vi "V50_OfficeReport.vi"(1 "Enable":bool=TRUE, 2 "blockFabric":variant, 3 "blockRange":variant, 4 "blockResults":variant, 5 "blockSample":variant, 6 "blockShotTbl":variant, 7 "error in (no error)":errorcluster, 8 "blockThreat":variant, 10 "method":variant, 11 "projName":variant, 12 "projNum":variant, 13 "recNum":variant, 14 "remark":variant, 15 "standard":variant) -> (27 "error out":errorcluster)   [LabVIEW 2010]
doc: "Allows you to configure Word and Excel reports using templates. You can use basic templates that the Report Generation Toolkit includes or you can create templates in Word and Excel.\n--------------------\n\nThis Express VI is configured as follows:\n\nTemplate Type: Custom Report for Excel\nDestination: Open in Microsoft Office"
uses:
  <vilib>/addons/_office/MSOfficeReportShared.llb/ex_RGT_Block State Information.ctl
  <vilib>/addons/_office/MSOfficeReportShared.llb/ex_RGT_Value Source.ctl
  <vilib>/addons/_office/MSOfficeReportShared.llb/ex_RGT_Input Appearance In Report.ctl
  <vilib>/addons/_office/MSOfficeReportShared.llb/ex_RGT_System Defined Value.ctl
  <vilib>/addons/_office/NI_ReportGenerationToolkit.lvlib
panel:
  in  "Template":u16(ring)=2 items=["Basic Excel Template", "Basic Word Template", "Custom Excel Template", "Custom Word Template"]
  in  "Path to Save Report":path=path "C:/Documents and Settings/krausdj/My Documents/LabVIEW Data/testReport.xls"
  in  "Bkm19":variant
  in  "Bkm18":variant
  in  "Printer Settings":T1={"Printer Name"="", "Number of Copies"=1}
  in  "standard":variant
  in  "remark":variant
  in  "projNum":variant
  in  "projName":variant
  in  "Date":variant=variant(string "10/31/2006")
  out "Saved Report Path":path
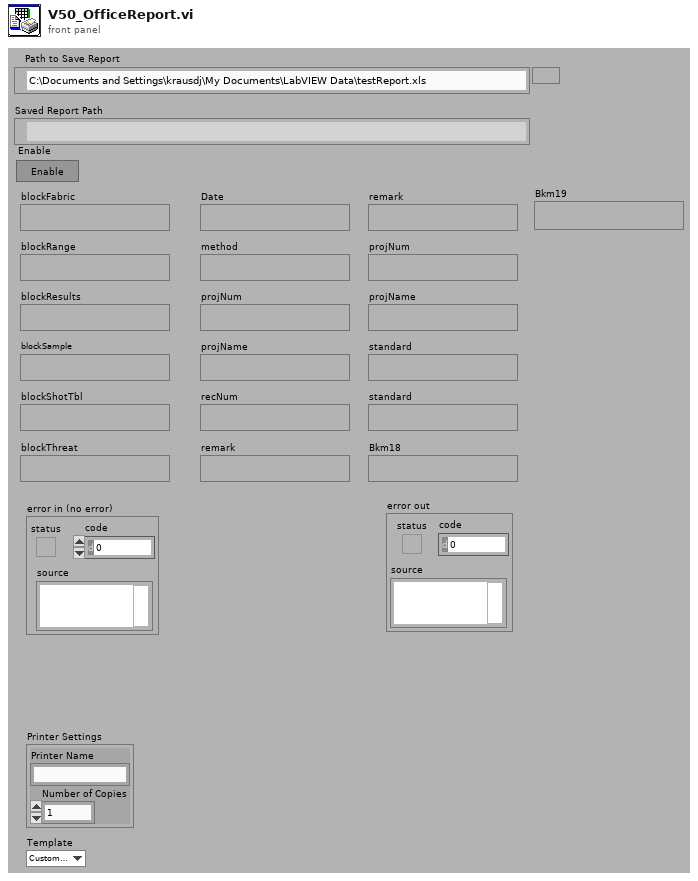
[diagram p1: front panel]
types:
  T1 = cluster{"Printer Name":string, "Number of Copies":i16}
  T2 = typedef "NI_ReportGenerationToolkit.lvlib/ex_RGT_Block State Information.ctl" = cluster{"Bookmark":string, "Value Source":T3, "Input Appearance in Report":T4, "Fixed Value":string, "System Defined Value":T5}
  T3 = typedef "NI_ReportGenerationToolkit.lvlib/ex_RGT_Value Source.ctl" = u16
  T4 = typedef "NI_ReportGenerationToolkit.lvlib/ex_RGT_Input Appearance In Report.ctl" = u16
  T5 = typedef "NI_ReportGenerationToolkit.lvlib/ex_RGT_System Defined Value.ctl" = u16
  T6 = enum16{"overwrite & backup", "next avail", "overwrite"}
  T7 = cluster{"HLP_Date Type":u16, "HLP_MDY":u16, "HLP_year":u16}
  T8 = cluster{"HLP_Time Type":u16, "HLP_Hour Type":u16, "HLP_HMS":u16}
  T9 = cluster{"format string for bookmark as Date":string, "format string for bookmark as Time":string}
  T10 = cluster{"BookMark/NamedCell":string, "Data":variant}
  T11 = cluster{"BookMark/NamedCell":string, "Data":variant}[]
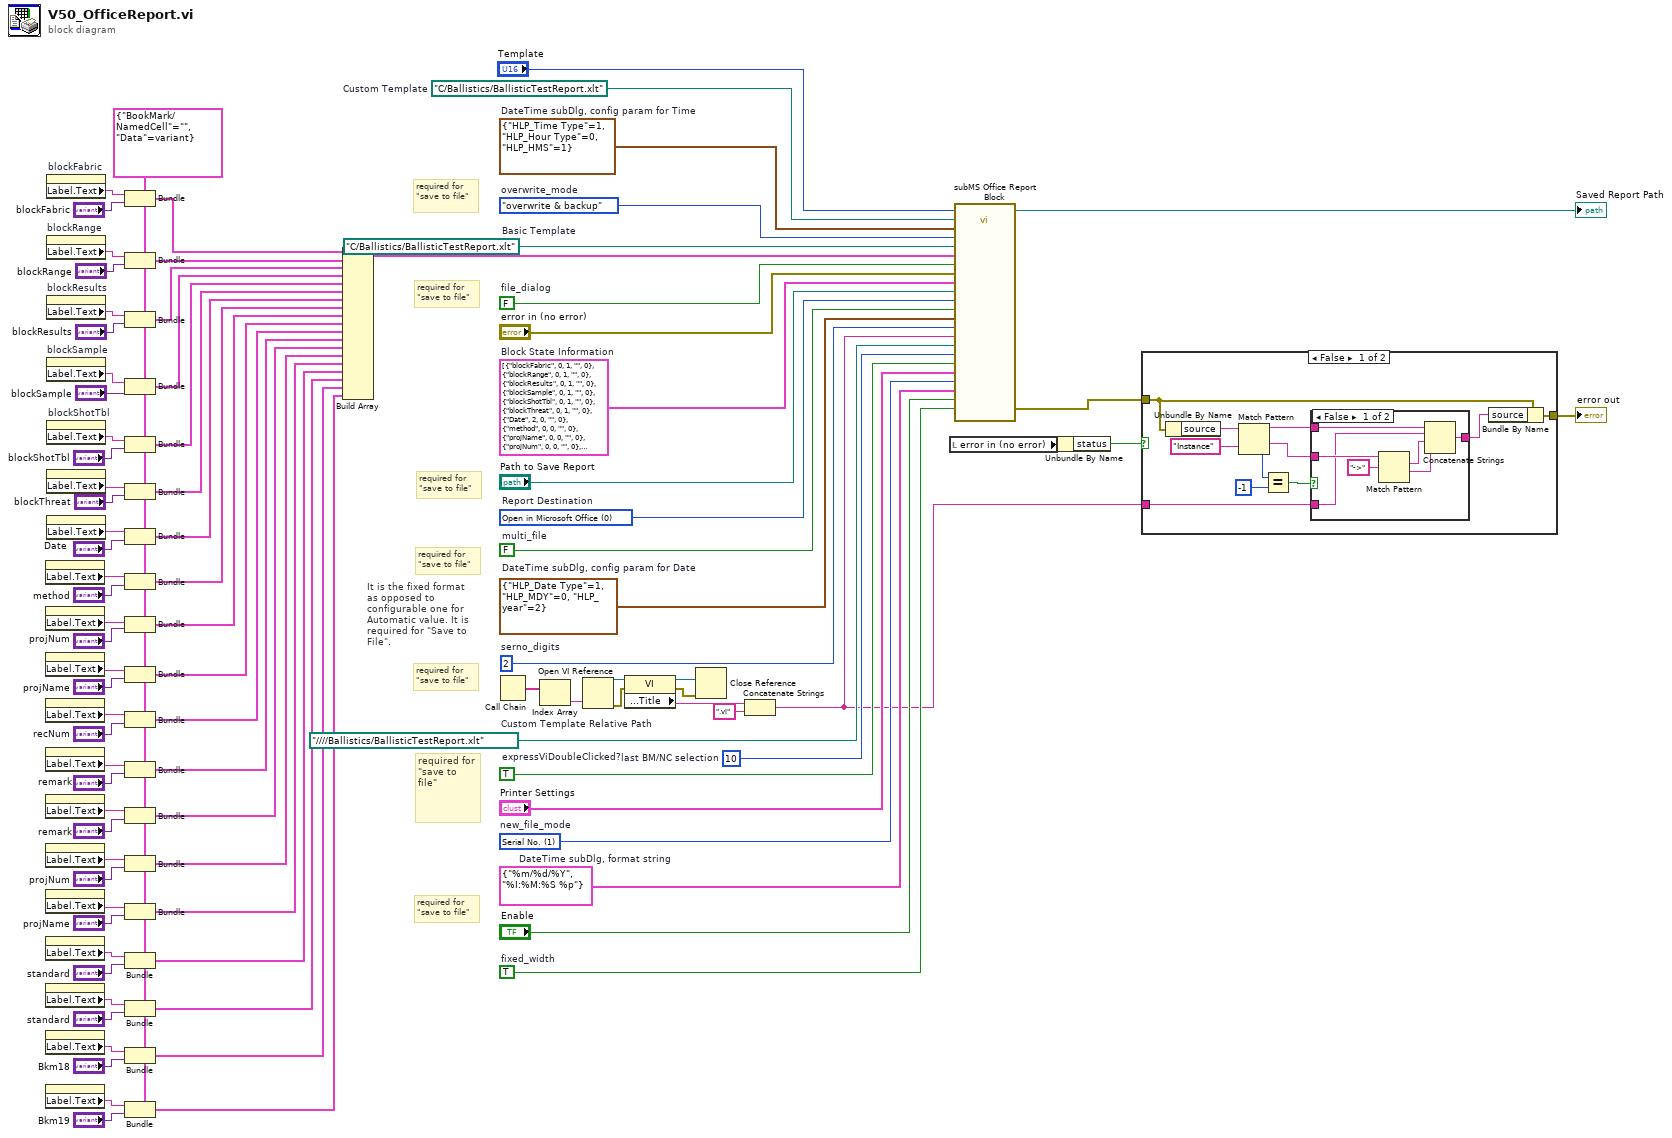
[diagram p0: block diagram]
diagram:
  w10 = path "../../../../Ballistics/BallisticTestReport.xlt"  # Custom Template Relative Path
  w18 = T2[] [{"Bookmark"="blockFabric", "Value Source"=0, "Input Appearance in Report"=1, "Fixed Value"="", "System Defined Value"=0}, {"Bookmark"="blockRange", "Value Source"=0, "Input Appearance in Report"=1, "Fixed Value"="", "System Defined Value"=0}, {"Bookmark"="blockResults", "Value Source"=0, "Input Appearance in Report"=1, "Fixed Value"="", "System Defined Value"=0}, {"Bookmark"="blockSample", "Value Source"=0, "Input Appearance in Report"=1, "Fixed Value"="", "System Defined Value"=0}, {"Bookmark"="blockShotTbl", "Value Source"=0, "Input Appearance in Report"=1, "Fixed Value"="", "System Defined Value"=0}, {"Bookmark"="blockThreat", "Value Source"=0, "Input Appearance in Report"=1, "Fixed Value"="", "System Defined Value"=0}, {"Bookmark"="Date", "Value Source"=2, "Input Appearance in Report"=0, "Fixed Value"="", "System Defined Value"=0}, {"Bookmark"="method", "Value Source"=0, "Input Appearance in Report"=0, "Fixed Value"="", "System Defined Value"=0}, {"Bookmark"="projName", "Value Source"=0, "Input Appearance in Report"=0, "Fixed Value"="", "System Defined Value"=0}, {"Bookmark"="projNum", "Value Source"=0, "Input Appearance in Report"=0, "Fixed Value"="", "System Defined Value"=0}, {"Bookmark"="recNum", "Value Source"=0, "Input Appearance in Report"=0, "Fixed Value"="", "System Defined Value"=0}, {"Bookmark"="remark", "Value Source"=0, "Input Appearance in Report"=0, "Fixed Value"="", "System Defined Value"=0}, {"Bookmark"="standard", "Value Source"=0, "Input Appearance in Report"=0, "Fixed Value"="", "System Defined Value"=0}]  # Block State Information
  w21 = T6."overwrite & backup"  # overwrite_mode
  w22 = 10  # last BM/NC selection
  w23 = T7 {"HLP_Date Type"=1, "HLP_MDY"=0, "HLP_year"=2}  # DateTime subDlg, config param for Date
  w24 = T8 {"HLP_Time Type"=1, "HLP_Hour Type"=0, "HLP_HMS"=1}  # DateTime subDlg, config param for Time
  w26 = T9 {"format string for bookmark as Date"="%m/%d/%Y", "format string for bookmark as Time"="%I:%M:%S %p"}  # DateTime subDlg, format string
  w20 = u16 0 items=["Open in Microsoft Office", "Print to Printer", "Save to File"]  # Report Destination
  w19 = TRUE  # expressViDoubleClicked?
  w79 = path "C:/Ballistics/BallisticTestReport.xlt"  # Custom Template
  w73 = u16 1 items=["Date & Time", "Serial No.", "Both"]  # new_file_mode
  w74 = TRUE  # fixed_width
  w75 = 2  # serno_digits
  w76 = FALSE  # multi_file
  w27 = FALSE  # file_dialog
  w29 = T10 {"BookMark/NamedCell"="", "Data"=variant} ("cluster")
  w78 = path "C:/Ballistics/BallisticTestReport.xlt"  # Basic Template
  # "It is the fixed format as opposed to configurable one for Automatic value. It is required for \"Save to File\"."
  # "required for \n\"save to file\""
  # "required for \n\"save to file\""
  # "required for \n\"save to file\""
  # "required for \n\"save to file\""
  # "required for \n\"save to file\""
  # "required for \n\"save to file\""
  # "required for \n\"save to file\""
  n1 = property on="method" class="LVVar"() -> ("Label.Text"=w68:string)  [unwired: 2 in, 2 out]
  n2 = property on="projNum" class="LVVar"() -> ("Label.Text"=w66:string)  [unwired: 2 in, 2 out]
  n3 = property on="projName" class="LVVar"() -> ("Label.Text"=w64:string)  [unwired: 2 in, 2 out]
  n4 = property on="recNum" class="LVVar"() -> ("Label.Text"=w62:string)  [unwired: 2 in, 2 out]
  n5 = property on="remark" class="LVVar"() -> ("Label.Text"=w60:string)  [unwired: 2 in, 2 out]
  n6 = property on="remark" class="LVVar"() -> ("Label.Text"=w58:string)  [unwired: 2 in, 2 out]
  n7 = property on="projNum" class="LVVar"() -> ("Label.Text"=w56:string)  [unwired: 2 in, 2 out]
  n8 = property on="projName" class="LVVar"() -> ("Label.Text"=w54:string)  [unwired: 2 in, 2 out]
  n9 = property on="standard" class="LVVar"() -> ("Label.Text"=w52:string)  [unwired: 2 in, 2 out]
  n10 = property on="standard" class="LVVar"() -> ("Label.Text"=w50:string)  [unwired: 2 in, 2 out]
  n11 = property on="Bkm18" class="LVVar"() -> ("Label.Text"=w34:string)  [unwired: 2 in, 2 out]
  n12 = property on="Bkm19" class="LVVar"() -> ("Label.Text"=w33:string)  [unwired: 2 in, 2 out]
  n13 = property on="blockFabric" class="LVVar"() -> ("Label.Text"=w94:string)  [unwired: 2 in, 2 out]
  n14 = property on="blockRange" class="LVVar"() -> ("Label.Text"=w92:string)  [unwired: 2 in, 2 out]
  n15 = property on="blockResults" class="LVVar"() -> ("Label.Text"=w90:string)  [unwired: 2 in, 2 out]
  n16 = property on="blockSample" class="LVVar"() -> ("Label.Text"=w88:string)  [unwired: 2 in, 2 out]
  n17 = property on="blockShotTbl" class="LVVar"() -> ("Label.Text"=w86:string)  [unwired: 2 in, 2 out]
  n18 = property on="blockThreat" class="LVVar"() -> ("Label.Text"=w72:string)  [unwired: 2 in, 2 out]
  n19 = property on="Date" class="LVVar"() -> ("Label.Text"=w70:string)  [unwired: 2 in, 2 out]
  n20 = Bundle(cluster=w29, "BookMark/NamedCell"=w94, "Data"="blockFabric") -> (w84:T10)
  n21 = Bundle(cluster=w29, "BookMark/NamedCell"=w92, "Data"="blockRange") -> (w83:T10)
  n22 = Bundle(cluster=w29, "BookMark/NamedCell"=w90, "Data"="blockResults") -> (w82:T10)
  n23 = Bundle(cluster=w29, "BookMark/NamedCell"=w88, "Data"="blockSample") -> (w81:T10)
  n24 = Bundle(cluster=w29, "BookMark/NamedCell"=w86, "Data"="blockShotTbl") -> (w80:T10)
  n25 = Bundle(cluster=w29, "BookMark/NamedCell"=w72, "Data"="blockThreat") -> (w48:T10)
  n26 = Bundle(cluster=w29, "BookMark/NamedCell"=w70, "Data"="Date") -> (w47:T10)
  n27 = Bundle(cluster=w29, "BookMark/NamedCell"=w68, "Data"="method") -> (w46:T10)
  n28 = Bundle(cluster=w29, "BookMark/NamedCell"=w66, "Data"="projNum") -> (w45:T10)
  n29 = Bundle(cluster=w29, "BookMark/NamedCell"=w64, "Data"="projName") -> (w44:T10)
  n30 = Bundle(cluster=w29, "BookMark/NamedCell"=w62, "Data"="recNum") -> (w43:T10)
  n31 = Bundle(cluster=w29, "BookMark/NamedCell"=w60, "Data"="remark") -> (w42:T10)
  n32 = Bundle(cluster=w29, "BookMark/NamedCell"=w58, "Data"="remark") -> (w41:T10)
  n33 = Bundle(cluster=w29, "BookMark/NamedCell"=w56, "Data"="projNum") -> (w40:T10)
  n34 = Bundle(cluster=w29, "BookMark/NamedCell"=w54, "Data"="projName") -> (w39:T10)
  n35 = Bundle(cluster=w29, "BookMark/NamedCell"=w52, "Data"="standard") -> (w38:T10)
  n36 = Bundle(cluster=w29, "BookMark/NamedCell"=w50, "Data"="standard") -> (w37:T10)
  n37 = Bundle(cluster=w29, "BookMark/NamedCell"=w34, "Data"="Bkm18") -> (w31:T10)
  n38 = Bundle(cluster=w29, "BookMark/NamedCell"=w33, "Data"="Bkm19") -> (w30:T10)
  n39 = Build Array(w84, w83, w82, w81, w80, w48, w47, w46, w45, w44, w43, w42, w41, w40, w39, w38, w37, w31, w30) -> (w77:T11)
  n40 = Call Chain() -> (call chain=w9:string[])
  n41 = Index Array(array=w9) -> (element=w8:string)  [unwired: 1 in]
  n42 = Open VI Reference(vi path=w8) -> (vi reference=w7:refnum<vi>, error out=w6:errorcluster)  [unwired: 5 in]
  n43 = property class="VI"(reference=w7, error in=w6) -> (reference out=w4:refnum<vi>, error out=w5:errorcluster, "Front Panel Window:Title"=w3:string)
  n44 = Close Reference(reference=w4, error in (no error)=w5) -> ()  [unwired: 1 out]
  n45 = Concatenate Strings(w3, ".vi" ("string")) -> (w1:string)
  n46 = local read "error in (no error)"() -> (w12:errorcluster)
  n47 = call <vilib>:"subMS Office Report Block.vi"("Template"="Template", "Custom Template"=w79, "DateTime subDlg, config param for Time"=w24, "overwrite_mode"=w21, "Basic Template"=w78, "Template Data"=w77, "file_dialog"=w27, "error in (no error)"="error in (no error)", "fixed_width"=w74, "Block State Information"=w18, "Enable"="Enable", "Path to Save Report"="Path to Save Report", "DateTime subDlg, format string"=w26, "Report Destination"=w20, "new_file_mode"=w73, "multi_file"=w76, "Printer Settings"="Printer Settings", "DateTime subDlg, config param for Date"=w23, "expressViDoubleClicked?"=w19, "serno_digits"=w75, "last BM/NC selection"=w22, "Custom Template Relative Path"=w10, "Block Label"=w1) -> ("Saved Report Path"=→"Saved Report Path":path, "error out"=w13:errorcluster)  [unwired: 3 in]
  n48 = Unbundle By Name(w12) -> ("status"=w11:bool)
  n49 = case shown="False" w11 {
    tunnel: [w96 w114] -> w14
    tunnel: w13 -> [w97 w114]
    tunnel: w1 -> [w95 _]
    frame False {
      n50 = Unbundle By Name(w97) -> ("source"=w105:string)
      n51 = Match Pattern(string=w105, regular expression="Instance") -> (before substring=w100:string, after substring=w99:string, offset past match=w102:i32)  [unwired: 1 in, 1 out]
      n52 = Equal?(x=w102, y=-1) -> (x = y?=w103:bool)
      n53 = case shown="False" w103 {
        tunnel: [w107 w113] -> w98
        tunnel: w100 -> [w112 w113]
        tunnel: w99 -> [w110 _]
        tunnel: w95 -> [w106 _]
        frame False {
          n54 = Match Pattern(string=w110, regular expression="->") -> (match substring=w109:string, after substring=w108:string)  [unwired: 1 in, 2 out]
          n55 = Concatenate Strings(w112, w106, w109, w108) -> (w107:string)
        }
        frame True {
        }
      }
      n56 = Bundle By Name(cluster=w97, "source"=w98) -> (w96:errorcluster)
    }
    frame True {
    }
  }
  "error out" <- w14
